vi "Update.vi"(8 "error in (no error)":errorcluster, 11 "Mixer in":refnum<class "Transport.lvclass">) -> (0 "error out":errorcluster, 2 "Record":bool, 3 "Mixer out":refnum<class "Transport.lvclass">)   [LabVIEW 2020, in "Transport.lvclass"]
uses:
  Transport.lvclass
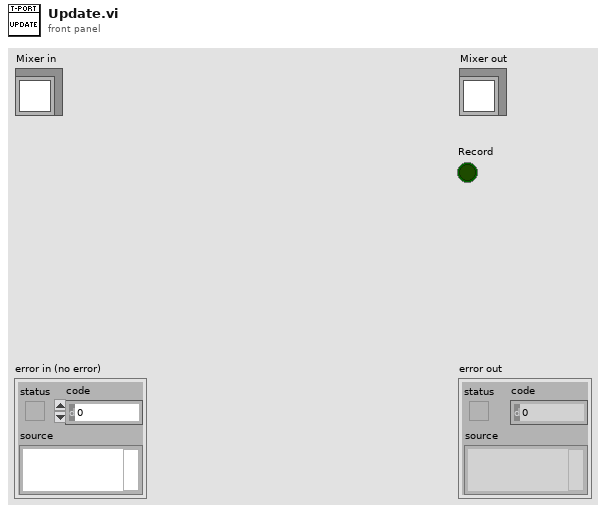
[diagram p1: front panel]
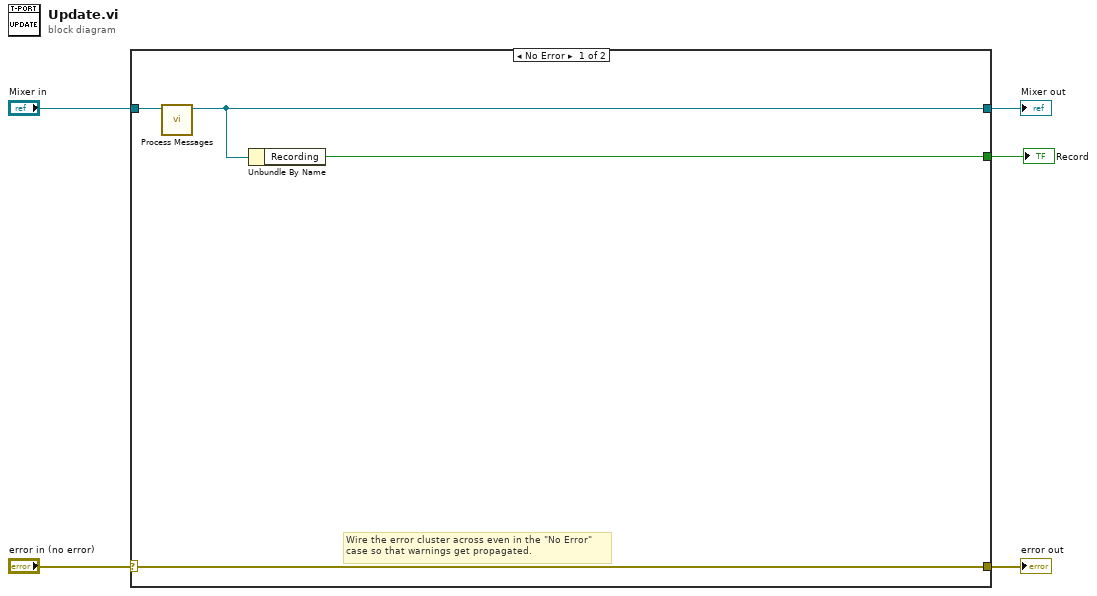
[diagram p0: block diagram]
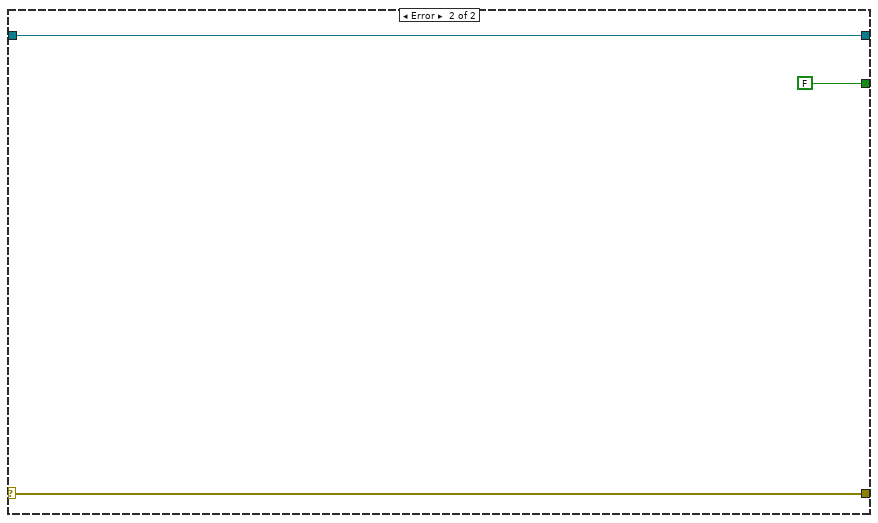
[diagram p2: hidden frame]
diagram:
  n1 = case shown="No Error" "error in (no error)" {
    selector: "error in (no error)" -> [w9 w12]
    tunnel: [w9 w12] -> w4
    tunnel: [w7 w11] -> w2
    tunnel: "Mixer in" -> [w8 w11]
    tunnel: [w6 FALSE ("Recording")] -> w1
    frame No Error {
      # "Wire the error cluster across even in the \"No Error\"\ncase so that warnings get propagated."
      n2 = call "Process Messages.vi"("Mixer in"=w8) -> ("Mixer out"=w7:refnum<class "Transport.lvclass">)  [unwired: 9 in, 1 out]
      n3 = Unbundle By Name(w7) -> ("Recording"=w6:bool)
    }
    frame Error {
    }
  }
  "error out" <- w4
  "Mixer out" <- w2
  "Record" <- w1
